vi "数据拼接.vi"(1 "数组":string[](array[string])) -> (0 "输出数据":i32[](array[numeric]))   [LabVIEW 2014]
panel:
  out "结果":i32[](array[numeric])
  out "波形图":i32[](graph)
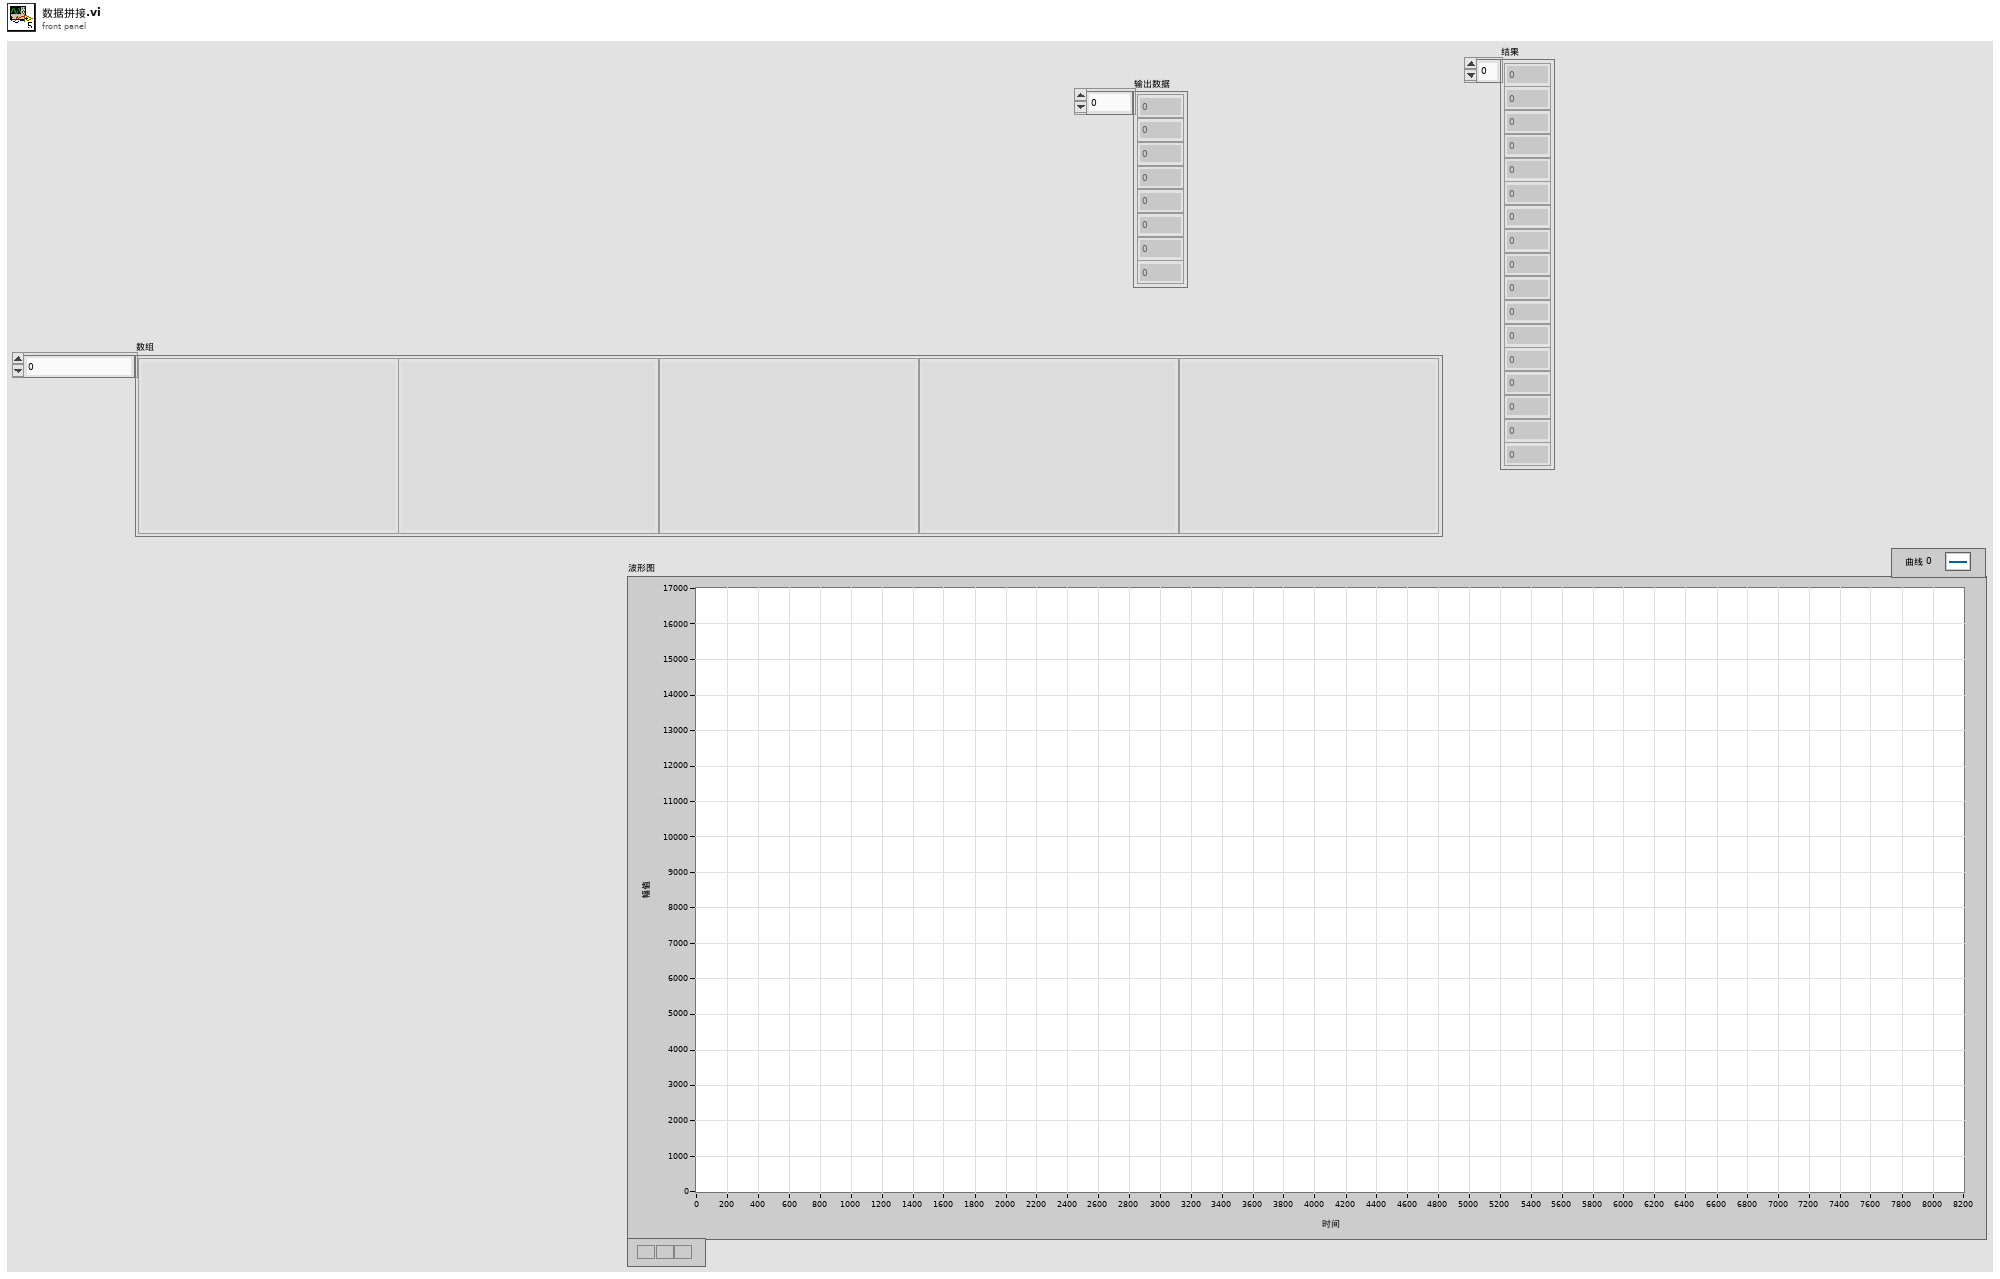
[diagram p1: front panel]
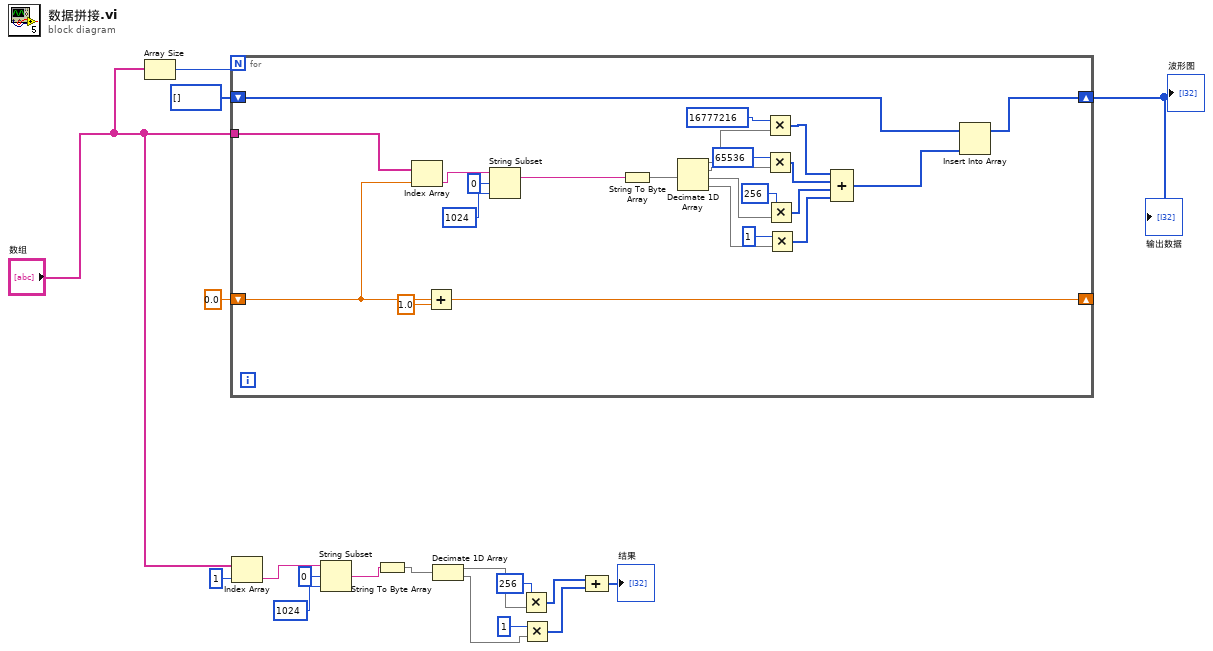
[diagram p0: block diagram]
diagram:
  n1 = Array Size(array="数组") -> (size(s)=w18:i32)
  n2 = for {
    N: w18 -> [_]
    tunnel: "数组" -> [w42]
    shift-right: [w33] -> w7
    shift-left: i32[] [] -> [w34]
    shift-right: [w27] -> _
    shift-left: 0.0 -> [w25]
    n3 = Index Array(array=w42, index=w25) -> (element=w31:string)
    n4 = Add(x=w25, y=1.0) -> (x+y=w27:dbl)
    n5 = String Subset(string=w31, offset (0)=0 ("偏移量(0)"), length (rest)=1024 ("长度（剩余）")) -> (substring=w28:string)
    n6 = String To Byte Array(string=w28) -> (unsigned byte array=w35:u8[])
    n7 = Decimate 1D Array(w35) -> (w21:u8[], w22:u8[], w41:u8[], w40:u8[])
    n8 = Multiply(x=u32 16777216, y=w21) -> (x*y=w19:u32[])
    n9 = Multiply(x=u32 65536, y=w22) -> (x*y=w24:u32[])
    n10 = Multiply(x=256, y=w41) -> (x*y=w36:i32[])
    n11 = Multiply(x=1, y=w40) -> (x*y=w37:i32[])
    n12 = Compound Arithmetic op=ADD(w19, w24, w36, w37) -> (w32:u32[])
    n13 = Insert Into Array(array=w34, new element=w32) -> (w33:i32[])  [unwired: 1 in]
  }
  "波形图" <- w7
  "输出数据" <- w7
  n14 = Index Array(array="数组", index=1 ("索引")) -> (element=w3:string)
  n15 = String Subset(string=w3, offset (0)=0 ("偏移量(0)"), length (rest)=1024 ("长度（剩余）")) -> (substring=w2:string)
  n16 = String To Byte Array(string=w2) -> (unsigned byte array=w10:u8[])
  n17 = Decimate 1D Array(w10) -> (w16:u8[], w15:u8[])
  n18 = Multiply(x=256, y=w16) -> (x*y=w11:i32[])
  n19 = Multiply(x=1, y=w15) -> (x*y=w12:i32[])
  n20 = Compound Arithmetic op=ADD(w11, w12) -> (→"结果":i32[])
